vi "Get Trigger ID.vi"(11 "TimerDRV in":refnum<class "TimerDRV.lvclass">) -> (2 "Trigger ID":u8, 3 "TimerDRV out":refnum<class "TimerDRV.lvclass">)   [LabVIEW 2019, in "TimingDRV Engine.lvlib" / "TimerDRV.lvclass"]
uses:
  TimerDRV.lvclass
  TimerDRV.lvclass/TimerDRV.ctl
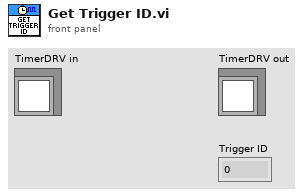
[diagram p1: front panel]
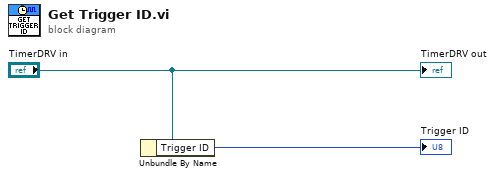
[diagram p0: block diagram]
diagram:
  n1 = Unbundle By Name("TimerDRV in") -> ("Trigger ID"=→"Trigger ID":u8)
  "TimerDRV out" <- "TimerDRV in"
